vi "Select Display Screen.vi"(8 "error in (no error)":errorcluster, 10 "Screen Home":u16(ring) items=["Home Screen", "Home Large Reading", "Reading Sheet", "Graph Screen", "Histogram", "Functions Swipe", "Graph Swipe", "Secondary Swipe", "Settings Swipe", "Statistics Swipe", "User Swipe", "Processing Screen"], 11 "VISA resource name":refnum<visa-resource-name>) -> (0 "error out":errorcluster, 3 "VISA resource name out":refnum<visa-resource-name>)   [LabVIEW 2023, in "Keithley DMM6500 DAQ6500 Series.lvlib"]
doc: "Enables or disables the display on the front of the instrument. Disabling the display can result in faster measurements."
uses:
  <instrlib>/Keithley DMM6500 DAQ6500 Series/Keithley DMM6500 DAQ6500 Series.lvlib
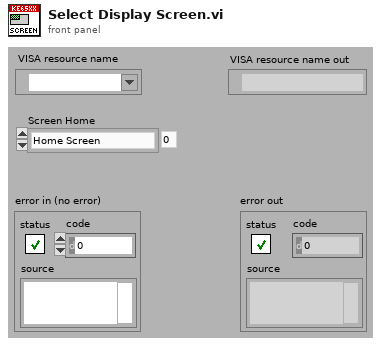
[diagram p1: front panel]
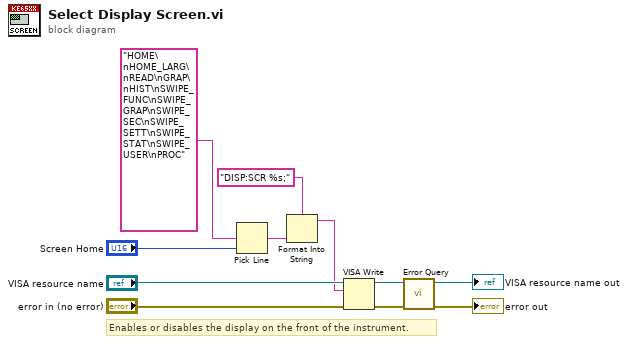
[diagram p0: block diagram]
diagram:
  # "Enables or disables the display on the front of the instrument."
  n1 = Pick Line(multi-line string="HOME\nHOME_LARG\nREAD\nGRAP\nHIST\nSWIPE_FUNC\nSWIPE_GRAP\nSWIPE_SEC\nSWIPE_SETT\nSWIPE_STAT\nSWIPE_USER\nPROC", line index="Screen Home") -> (output string=w5:string)  [unwired: 1 in]
  n2 = Format Into String(format string="DISP:SCR %s;", w5) -> (resulting string=w8:string)  [unwired: 2 in, 1 out]
  n3 = VISA Write(VISA resource name="VISA resource name", write buffer=w8, error in (no error)="error in (no error)") -> (VISA resource name out=w4:refnum<visa-resource-name>, error out=w2:errorcluster)  [unwired: 1 out]
  n4 = call <instrlib>:"Error Query.vi"("error in (no error)"=w2, "VISA resource name"=w4) -> ("error out"=→"error out":errorcluster, "VISA resource name out"=→"VISA resource name out":refnum<visa-resource-name>)  [unwired: 6 in, 2 out]
